vi "RakeLocations.vi"(9 "Rake Spacing":dbl, 10 "Rake Points (n)":u32, 11 "Rake Centre Position":dbl) -> (3 "Locations":dbl[](array[numeric]))   [LabVIEW 2011]
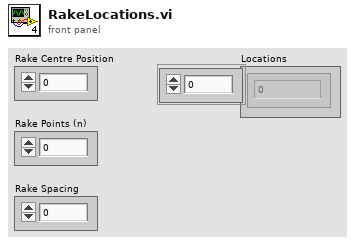
[diagram p1: front panel]
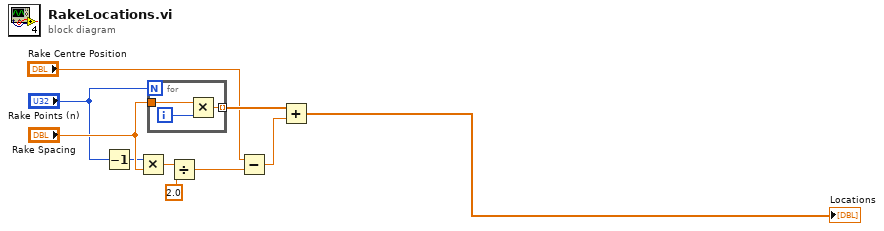
[diagram p0: block diagram]
diagram:
  n1 = Decrement(x="Rake Points (n)") -> (x-1=w4:u32)
  n2 = Multiply(x=w4, y="Rake Spacing") -> (x*y=w1:dbl)
  n3 = for {
    N: "Rake Points (n)" -> [_]
    tunnel: "Rake Spacing" -> [w12]
    tunnel: [w11] -> w9 mode=indexing
    i -> [w13]
    n4 = Multiply(x=w12, y=w13) -> (x*y=w11:dbl)
  }
  n5 = Divide(x=w1, y=2.0) -> (x/y=w5:dbl)
  n6 = Subtract(x="Rake Centre Position", y=w5) -> (x-y=w10:dbl)
  n7 = Add(x=w9, y=w10) -> (x+y=→"Locations":dbl[])
